vi "Read (0D U8).vi"(8 "error in (no error)":errorcluster, 9 "offset (0)":u64 format="%d bytes", 10 "value in":u8, 11 "Pointer in":refnum<class "Pointer.lvclass">) -> (0 "error out":errorcluster, 1 "offset out":u64 format="%d bytes", 2 "value out":u8, 3 "Pointer out":refnum<class "Pointer.lvclass">)   [LabVIEW 2016, in "Memory Manager.lvlib" / "Pointer.lvclass"]
doc: "Reads the contents of the address specified by <b>pointer + offset</b> into <b>value</b>.\n\n<b>Note:</b> This VI is <b>safe</b>.\n\nSafe means that this function evaluates the size parameter of <b>pointer</b> to ensure that is inbounds of allocated memory before peforming a memory read/write. Reading/writing more data to a pointer than it has allocated can corrupt or crash LabVIEW."
uses:
  Pointer.lvclass
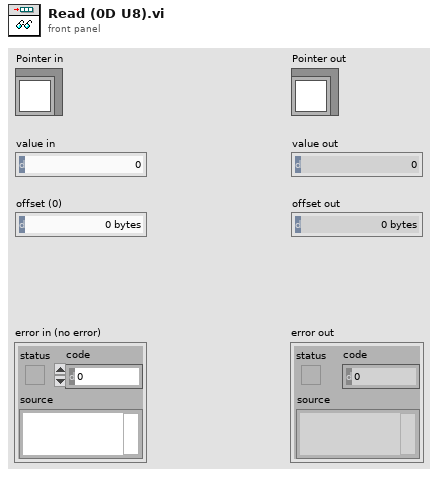
[diagram p1: front panel]
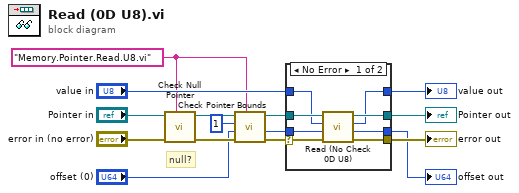
[diagram p0: block diagram]
diagram:
  w4 = "Memory.Pointer.Read.U8.vi" ("source vi name")
  # "null?"
  n1 = call "Check Null Pointer.vi"("source vi name"=w4, "error in (no error)"="error in (no error)", "Pointer in"="Pointer in") -> ("error out"=w6:errorcluster, "Pointer out"=w7:refnum<class "Pointer.lvclass">)  [unwired: 7 in]
  n2 = call "Check Pointer Bounds.vi"("source vi name"=w4, "error in (no error)"=w6, "offset (0)"="offset (0)", "size"=u64 1 ("y"), "Pointer in"=w7) -> ("error out"=w13:errorcluster, "offset out"=w2:u64, "Pointer out"=w15:refnum<class "Pointer.lvclass">)  [unwired: 3 in, 1 out]
  n3 = case shown="No Error" w13 {
    selector: w13 -> [w19 w25]
    tunnel: w15 -> [w23 w27]
    tunnel: [w22 w27] -> w9
    tunnel: [w21 w26] -> w11
    tunnel: "value in" -> [w20 w26]
    tunnel: [w18 w25] -> w10
    tunnel: w2 -> [w17 w24]
    tunnel: [w16 w24] -> w1
    frame No Error {
      n4 = call "Read (No Check 0D U8).vi"("error in (no error)"=w19, "offset (0)"=w17, "value in"=w20, "Pointer in"=w23) -> ("error out"=w18:errorcluster, "offset out"=w16:u64, "value out"=w21:u8, "Pointer out"=w22:refnum<class "Pointer.lvclass">)  [unwired: 4 in]
    }
    frame Error {
    }
  }
  "error out" <- w10
  "Pointer out" <- w9
  "value out" <- w11
  "offset out" <- w1
